vi "Read operation (0_open).vi"(8 "error in (no error)":errorcluster, 11 "Write_to_file in":refnum<class "Write_to_file.lvclass">) -> (0 "error out":errorcluster, 2 "operation (0:open)":T1(ring)=enum."replace or create", 3 "Write_to_file out":refnum<class "Write_to_file.lvclass">)   [LabVIEW 2019, in "Write_to_file.lvclass"]
uses:
  Write_to_file.lvclass
  Write_to_file.lvclass/Write_to_file.ctl
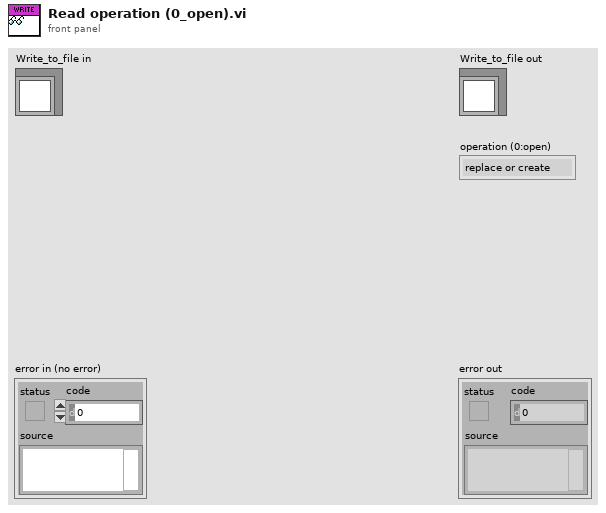
[diagram p1: front panel]
types:
  T1 = enum16{"open", "replace", "create", "open or create", "replace or create", "replace or create with confirmation"}
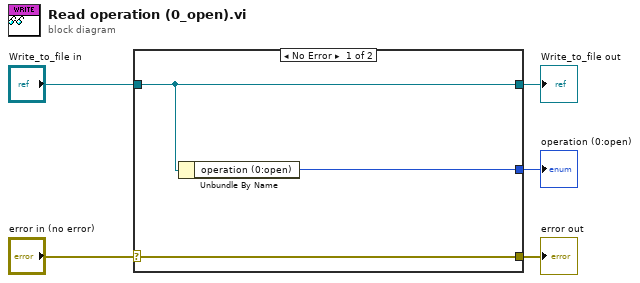
[diagram p0: block diagram]
diagram:
  n1 = case shown="No Error" "error in (no error)" {
    selector: "error in (no error)" -> [w8 w9]
    tunnel: [w8 w9] -> w4
    tunnel: [w7 w10] -> w2
    tunnel: "Write_to_file in" -> [w7 w10]
    tunnel: [w6 _] -> w1
    frame No Error {
      n2 = Unbundle By Name(w7) -> ("operation (0:open)"=w6:T1)
    }
    frame Error {
    }
  }
  "error out" <- w4
  "Write_to_file out" <- w2
  "operation (0:open)" <- w1
